vi "Waveform Manipulation.vi"() -> ()   [LabVIEW 2018]
uses:
  AnalysisSupport.lvlib
panel:
  out "Waveform Chart 4":dynamicdata(graph)
  out "Waveform Chart 3":dynamicdata(graph)
  out "Waveform Chart 2":dynamicdata(graph)
  out "Waveform Chart":dynamicdata(graph)
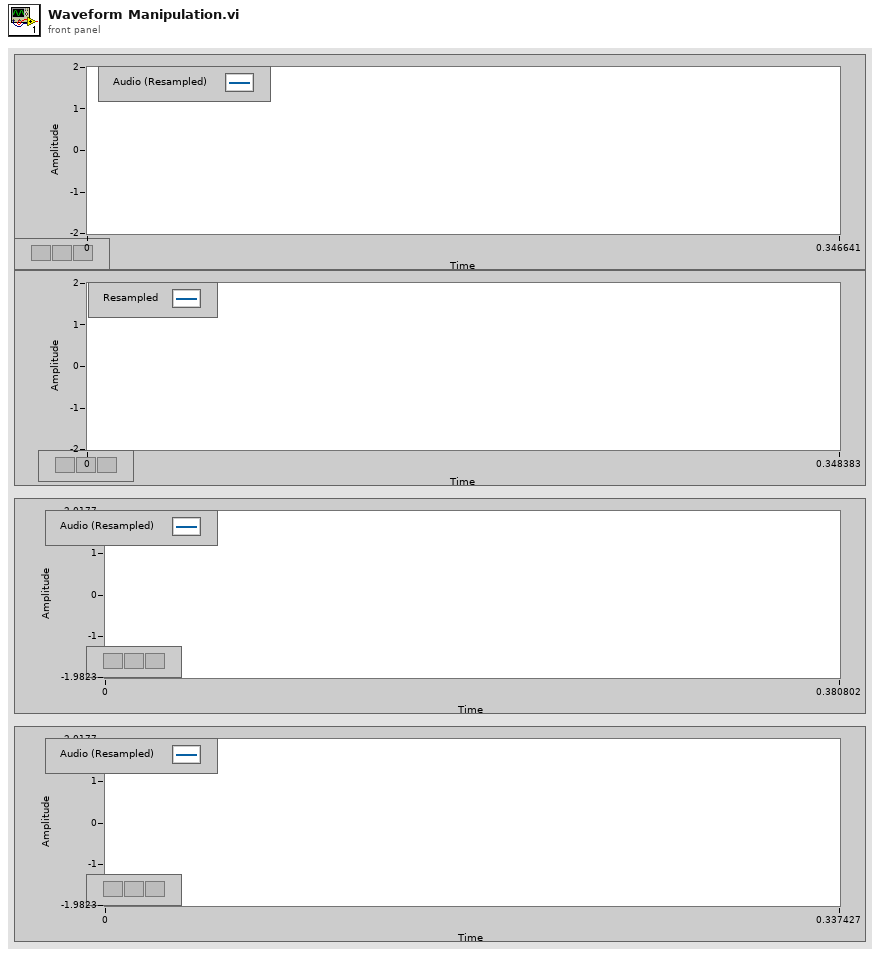
[diagram p1: front panel]
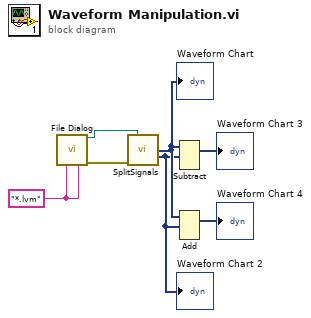
[diagram p0: block diagram]
diagram:
  w5 = "*.lvm" ("pattern (all files)")
  n1 = call "File Dialog"("pattern (all files)"=w5, "pattern label"=w5) -> ("selected path"=w6:path, "error out"=w7:errorcluster)  [unwired: 10 in, 2 out]
  n2 = call "SplitSignals.vi"("Filename"=w6, "Error In"=w7) -> ("Audio"=w3:dynamicdata, "SPL"=w2:dynamicdata)  [unwired: 6 in, 6 out]
  "Waveform Chart" <- w3
  "Waveform Chart 2" <- w2
  n3 = Subtract(1:w2, 2:w3) -> (0:→"Waveform Chart 3":dynamicdata)  [unwired: 1 in, 1 out]
  n4 = Add(1:w2, 2:w3) -> (0:→"Waveform Chart 4":dynamicdata)  [unwired: 1 in, 1 out]
